vi "Set pos scrollbar limits.vi"(8 "error in (no error)":errorcluster, 9 "Min frame (unity-based)":u32, 10 "Max frame (unity-based)":u32) -> (0 "error out":errorcluster)   [LabVIEW 2020]
uses:
  Globals/gl_Time series viewer globals.vi
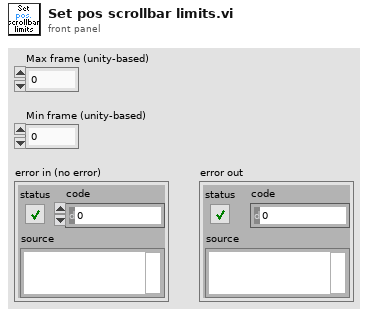
[diagram p1: front panel]
types:
  T1 = typedef "Time series viewer refs.ctl" = cluster{"This VI":refnum<vi>, "Image control":refnum<vi>, "AVI Mode ind":refnum<vi>, "Play":refnum<vi>, "Stop":refnum<vi>, "Back":refnum<vi>, "Scrollbar":refnum<vi>, "Video length info":refnum<vi>, "Expected speed values":refnum<vi>, "Intensity":refnum<vi>, "Path":refnum<vi>, "Selection sliders":refnum<vi>, "Speed Graph ref":refnum<vi>, "Frame rate set (fps)":refnum<vi>, "Number of rows to generate":refnum<vi>, "VL Image Array":refnum<vi>, "Image Scrollbar":refnum<vi>, "Channel to load":refnum<vi>, "Colour":refnum<vi>}
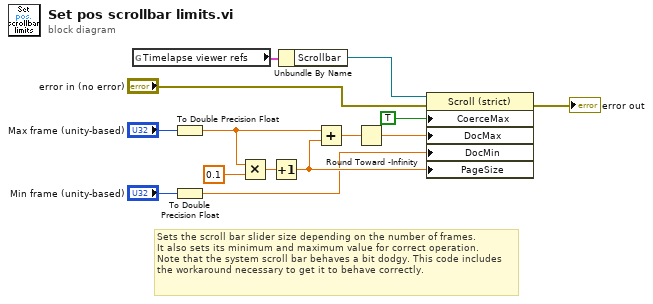
[diagram p0: block diagram]
diagram:
  # "Sets the scroll bar slider size depending on the number of frames.\nIt also sets its minimum and maximum value for correct operation.\nNote that the system scroll bar behaves a bit dodgy. This code includes the workaround necessary to get it to behave correctly."
  n1 = global read "gl_Time series viewer globals.vi" "Timelapse viewer refs"() -> (w5:T1)
  n2 = To Double Precision Float(number="Max frame (unity-based)") -> (double precision float=w14:dbl)
  n3 = To Double Precision Float(number="Min frame (unity-based)") -> (double precision float=w6:dbl)
  n4 = Multiply(x=w14, y=0.1) -> (x*y=w9:dbl)
  n5 = Increment(x=w9) -> (x+1=w11:dbl)
  n6 = Unbundle By Name(w5) -> ("Scrollbar"=w4:refnum<vi>)
  n7 = Add(x=w14, y=w11) -> (x+y=w1:dbl)
  n8 = Round Toward -Infinity(1:w1) -> (0:w3:dbl)
  n9 = property on="Property Node" class="Scroll (strict)"(reference=w4, error in="error in (no error)", "CoerceMax"=TRUE ("Coerce Maximum Value"), "DocMax"=w3, "DocMin"=w6, "PageSize"=w11) -> (error out=→"error out":errorcluster)  [unwired: 1 out]
